vi "Replace Json Tag.vi"(9 "Part Number PCBA":string(combo), 10 "Type Product":string(combo)="PCBA", 11 "Parameter (Json) en entrée":string) -> (3 "Parameter (Json) en sortie":string)   [LabVIEW 2020, in "Library Commun.lvlib"]
uses:
  Commun VI/Library Commun.lvlib
  Class/JSON API/Variant JSON/Variant to JSON.vi
  Class/JSON API/JSON Value/Get Item by name array.vi
  Class/JSON API/JSON Value/JSON Value.lvclass
  Class/JSON API/Get Polymorphic/JSON GetSet.lvlib
  Class/JSON API/Variant JSON/Variant JSON.lvlib
panel:
  in  "Tableau":string[](array[string])=["<PathFW>", "<Path>", "<PathParameter>", "<PathLabel>", "<PathLog>"]
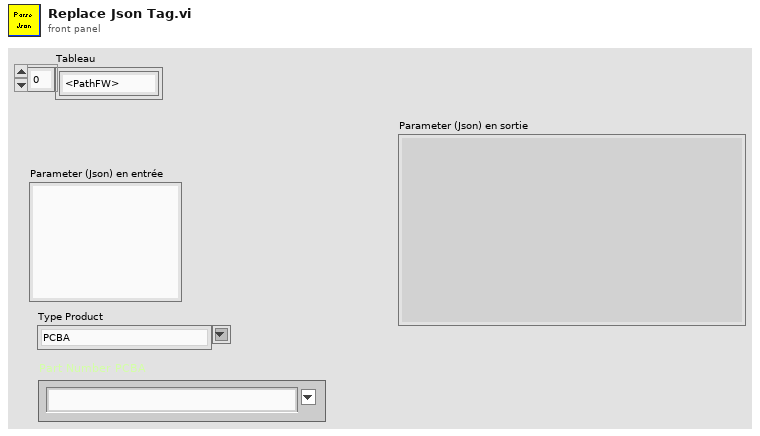
[diagram p1: front panel]
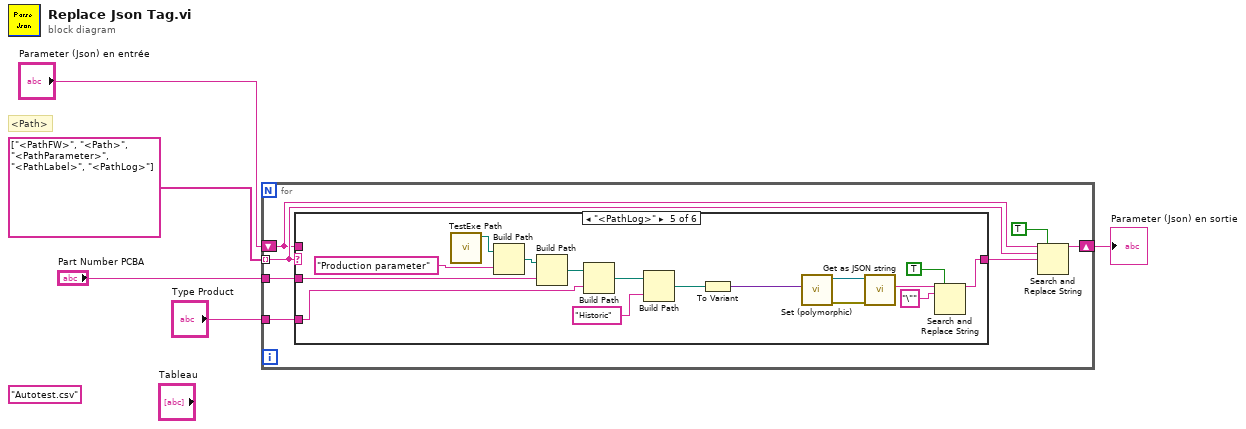
[diagram p0: block diagram]
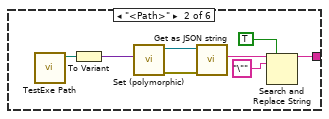
[diagram p3: hidden frame]
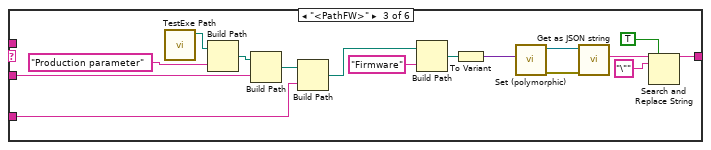
[diagram p4: hidden frame]
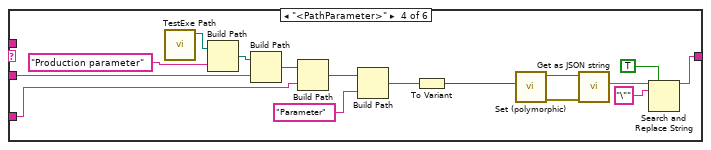
[diagram p5: hidden frame]
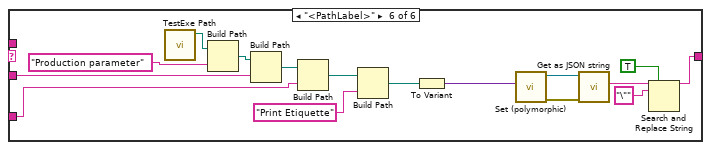
[diagram p6: hidden frame]
diagram:
  (unwired) "Autotest.csv" ("nom ou chemin relatif")
  # "<Path>"
  n1 = for {
    tunnel: string[] ["<PathFW>", "<Path>", "<PathParameter>", "<PathLabel>", "<PathLog>"] -> [w10] mode=indexing
    shift-right: [w11] -> w4
    shift-left: "Parameter (Json) en entrée" -> [w8]
    tunnel: "Part Number PCBA" -> [w7]
    tunnel: "Type Product" -> [w6]
    n2 = case shown="\"<PathLog>\"" w10 {
      selector: w10 -> [w13 _ _ _ _ _]
      tunnel: w8 -> [_ _ _ _ _ _]
      tunnel: [w13 w14 w24 w40 w56 w72] -> w9
      tunnel: w7 -> [_ _ w23 w39 w55 w71]
      tunnel: w6 -> [_ _ w22 w38 w54 w70]
      frame Default {
        # "膊膊"
      }
      frame "<Path>" {
        n3 = call "TestExe Path.vi"() -> ("Chemin Actuel"=w18:path)  [unwired: 9 in, 2 out]
        n4 = To Variant(anything=w18) -> (Variant=w21:variant)
        n5 = call-poly "Set (polymorphic).vi"("Variant"=w21) -> ("error out"=w19:errorcluster, "JSON Value out"=w20:refnum<class "JSON Value.lvclass">)  [unwired: 9 in]
        n6 = call "Get as JSON string.vi"("error in (no error)"=w19, "JSON Value in"=w20) -> ("<JSON>"=w15:string)  [unwired: 8 in, 1 out]
        n7 = Search and Replace String(replace all?=TRUE ("tout remplacer ? (F)"), input string=w15, search string="\"" ("chaîne recherchée")) -> (result string=w14:string)  [unwired: 5 in, 3 out]
      }
      frame "<PathFW>" {
        n8 = call "TestExe Path.vi"() -> ("Chemin Actuel"=w28:path)  [unwired: 9 in, 2 out]
        n9 = Build Path(base path=w28, name or relative path="Production parameter" ("nom ou chemin relatif")) -> (appended path=w29:path)
        n10 = Build Path(base path=w29, name or relative path=w23) -> (appended path=w30:path)
        n11 = Build Path(base path=w30, name or relative path=w22) -> (appended path=w31:path)
        n12 = Build Path(base path=w31, name or relative path="Firmware" ("nom ou chemin relatif")) -> (appended path=w25:path)
        n13 = To Variant(anything=w25) -> (Variant=w37:variant)
        n14 = call-poly "Set (polymorphic).vi"("Variant"=w37) -> ("error out"=w35:errorcluster, "JSON Value out"=w36:refnum<class "JSON Value.lvclass">)  [unwired: 9 in]
        n15 = call "Get as JSON string.vi"("error in (no error)"=w35, "JSON Value in"=w36) -> ("<JSON>"=w32:string)  [unwired: 8 in, 1 out]
        n16 = Search and Replace String(replace all?=TRUE ("tout remplacer ? (F)"), input string=w32, search string="\"" ("chaîne recherchée")) -> (result string=w24:string)  [unwired: 5 in, 3 out]
      }
      frame "<PathParameter>" {
        n17 = call "TestExe Path.vi"() -> ("Chemin Actuel"=w44:path)  [unwired: 9 in, 2 out]
        n18 = Build Path(base path=w44, name or relative path="Production parameter" ("nom ou chemin relatif")) -> (appended path=w45:path)
        n19 = Build Path(base path=w45, name or relative path=w39) -> (appended path=w46:path)
        n20 = Build Path(base path=w46, name or relative path=w38) -> (appended path=w47:path)
        n21 = Build Path(base path=w47, name or relative path="Parameter" ("nom ou chemin relatif")) -> (appended path=w41:path)
        n22 = To Variant(anything=w41) -> (Variant=w53:variant)
        n23 = call-poly "Set (polymorphic).vi"("Variant"=w53) -> ("error out"=w51:errorcluster, "JSON Value out"=w52:refnum<class "JSON Value.lvclass">)  [unwired: 9 in]
        n24 = call "Get as JSON string.vi"("error in (no error)"=w51, "JSON Value in"=w52) -> ("<JSON>"=w48:string)  [unwired: 8 in, 1 out]
        n25 = Search and Replace String(replace all?=TRUE ("tout remplacer ? (F)"), input string=w48, search string="\"" ("chaîne recherchée")) -> (result string=w40:string)  [unwired: 5 in, 3 out]
      }
      frame "<PathLog>" {
        n26 = call "TestExe Path.vi"() -> ("Chemin Actuel"=w60:path)  [unwired: 9 in, 2 out]
        n27 = Build Path(base path=w60, name or relative path="Production parameter" ("nom ou chemin relatif")) -> (appended path=w61:path)
        n28 = Build Path(base path=w61, name or relative path=w55) -> (appended path=w62:path)
        n29 = Build Path(base path=w62, name or relative path=w54) -> (appended path=w63:path)
        n30 = Build Path(base path=w63, name or relative path="Historic" ("nom ou chemin relatif")) -> (appended path=w57:path)
        n31 = To Variant(anything=w57) -> (Variant=w69:variant)
        n32 = call-poly "Set (polymorphic).vi"("Variant"=w69) -> ("error out"=w67:errorcluster, "JSON Value out"=w68:refnum<class "JSON Value.lvclass">)  [unwired: 9 in]
        n33 = call "Get as JSON string.vi"("error in (no error)"=w67, "JSON Value in"=w68) -> ("<JSON>"=w64:string)  [unwired: 8 in, 1 out]
        n34 = Search and Replace String(replace all?=TRUE ("tout remplacer ? (F)"), input string=w64, search string="\"" ("chaîne recherchée")) -> (result string=w56:string)  [unwired: 5 in, 3 out]
      }
      frame "<PathLabel>" {
        n35 = call "TestExe Path.vi"() -> ("Chemin Actuel"=w76:path)  [unwired: 9 in, 2 out]
        n36 = Build Path(base path=w76, name or relative path="Production parameter" ("nom ou chemin relatif")) -> (appended path=w77:path)
        n37 = Build Path(base path=w77, name or relative path=w71) -> (appended path=w78:path)
        n38 = Build Path(base path=w78, name or relative path=w70) -> (appended path=w79:path)
        n39 = Build Path(base path=w79, name or relative path="Print Etiquette" ("nom ou chemin relatif")) -> (appended path=w73:path)
        n40 = To Variant(anything=w73) -> (Variant=w85:variant)
        n41 = call-poly "Set (polymorphic).vi"("Variant"=w85) -> ("error out"=w83:errorcluster, "JSON Value out"=w84:refnum<class "JSON Value.lvclass">)  [unwired: 9 in]
        n42 = call "Get as JSON string.vi"("error in (no error)"=w83, "JSON Value in"=w84) -> ("<JSON>"=w80:string)  [unwired: 8 in, 1 out]
        n43 = Search and Replace String(replace all?=TRUE ("tout remplacer ? (F)"), input string=w80, search string="\"" ("chaîne recherchée")) -> (result string=w72:string)  [unwired: 5 in, 3 out]
      }
    }
    n44 = Search and Replace String(replace all?=TRUE ("tout remplacer ? (F)"), input string=w8, search string=w10, replace string=w9) -> (result string=w11:string)  [unwired: 4 in, 3 out]
  }
  "Parameter (Json) en sortie" <- w4
